vi "strange cluster.vi"(8 "Array In":T1(array[cluster]) {"Gauge" scale=0.0..100.0}, 11 "Cluster In":T2={"Gauge"=49.62882071738944, "Boolean def on"=TRUE, "My String"="abc", "Boolean def off"=FALSE, "Table"=[["1", "2", "3"], ["a", "b", "b"]], "Waveform Graph"={"t0"=timestamp(0 s since 1904-01-01), "dt"=0.001, "Y"=[0.0, 0.0634175857813252, 0.1265798623799041, 0.18923254844743084, 0.2511234141665813, 0.3120032966884148, 0.3716271032226454, 0.4297547977425003, 0.4861523673318466, 0.5405927642842268, 0.5928568201610591, 0.6427341281291522, 0.6900238900253773, 0.7345357247383564, 0.7760904346527414, 0.8145207270705094, 0.8496718877049362, 0.8814024035358785, 0.9095845325188363, 0.9341048178542484, 0.9548645447466428, 0.9717801378148127, 0.9847834975530967, 0.993822274489234, 0.9988600799350685, 0.9998766324816606, 0.9968678396490348, 0.9898458143618585, 0.9788388261847202, 0.9638911875133281, 0.9450630751798048, 0.9224302881902667, 0.8960839425699989, 0.8661301045447303, 0.8326893635347631, 0.7958963466810159, 0.7558991768574196, 0.7128588763516256, 0.6669487186147105, 0.6183535306896335, 0.5672689491267566, 0.5139006323819968, 0.458463432868368, 0.40118053199410575, 0.3422825416695715, 0.28200657590012973, 0.22059529620261753, 0.15829593468840908, 0.09535929874598903, 0.03203876133002422, -0.03141075907812785, -0.09473382473195789, -0.15767550697182214, -0.21998241252745737, -0.2814037036392598, -0.3416921078914828, -0.40060491369192236, -0.45790494739044835, -0.5133615281026551, -0.5667513963946633, -0.6178596130903338, -0.6664804245824388, -0.7124180911641828, -0.7554876750463428, -0.7955157848875944, -0.832341273840663, -0.8658158883040745, -0.8958048647677382, -0.9221874723495489, -0.944857498838849, -0.9637236782900093, -0.9787100584447116, -0.9897563065037406, -0.9968179520173057, -0.9998665659160451, -0.9988898749619699, -0.99389181115858, -0.9848924959212413, -0.9719281590715428, -0.9550509929817614, -0.934328942456612, -0.9098454311981998, -0.8816990259553703, -0.8500030397095515, -0.8148850754945864, -0.776486512687079, -0.7349619378353532, -0.6904785223184312, -0.6432153493404656, -0.593362692970051, -0.5411212521268765, -0.48670134259958137, -0.43032205034760956, -0.3722103494957459, -0.312600188572142, -0.251731548668498, -0.18984947731409485, -0.1272031019531499, -0.06404462699707955, -0.0006283184893772641], "attributes"=variant("NI_ChannelName"=variant(string "Sine"), "NI_ExpIsRelativeTime"=variant(bool TRUE), "NI_ExpStartTimeStamp"=variant(timestamp timestamp(3210167528.3009996 s since 1904-01-01)), "NI_ExpTimeStamp"=variant(timestamp timestamp(3210167528.3009996 s since 1904-01-01)), "NI_ExpXDimension"=variant(string "t"))}} {"Gauge" scale=0.0..100.0}) -> (0 "Array Out":T1(array[cluster]) {"Gauge" scale=0.0..100.0}, 3 "Cluster Out":T2={"Gauge"=49.62882071738944, "Boolean def on"=TRUE, "My String"="abc", "Boolean def off"=FALSE, "Table"=[["1", "2", "3"], ["a", "b", "b"]], "Waveform Graph"={"t0"=timestamp(0 s since 1904-01-01), "dt"=0.001, "Y"=[0.0, 0.0634175857813252, 0.1265798623799041, 0.18923254844743084, 0.2511234141665813, 0.3120032966884148, 0.3716271032226454, 0.4297547977425003, 0.4861523673318466, 0.5405927642842268, 0.5928568201610591, 0.6427341281291522, 0.6900238900253773, 0.7345357247383564, 0.7760904346527414, 0.8145207270705094, 0.8496718877049362, 0.8814024035358785, 0.9095845325188363, 0.9341048178542484, 0.9548645447466428, 0.9717801378148127, 0.9847834975530967, 0.993822274489234, 0.9988600799350685, 0.9998766324816606, 0.9968678396490348, 0.9898458143618585, 0.9788388261847202, 0.9638911875133281, 0.9450630751798048, 0.9224302881902667, 0.8960839425699989, 0.8661301045447303, 0.8326893635347631, 0.7958963466810159, 0.7558991768574196, 0.7128588763516256, 0.6669487186147105, 0.6183535306896335, 0.5672689491267566, 0.5139006323819968, 0.458463432868368, 0.40118053199410575, 0.3422825416695715, 0.28200657590012973, 0.22059529620261753, 0.15829593468840908, 0.09535929874598903, 0.03203876133002422, -0.03141075907812785, -0.09473382473195789, -0.15767550697182214, -0.21998241252745737, -0.2814037036392598, -0.3416921078914828, -0.40060491369192236, -0.45790494739044835, -0.5133615281026551, -0.5667513963946633, -0.6178596130903338, -0.6664804245824388, -0.7124180911641828, -0.7554876750463428, -0.7955157848875944, -0.832341273840663, -0.8658158883040745, -0.8958048647677382, -0.9221874723495489, -0.944857498838849, -0.9637236782900093, -0.9787100584447116, -0.9897563065037406, -0.9968179520173057, -0.9998665659160451, -0.9988898749619699, -0.99389181115858, -0.9848924959212413, -0.9719281590715428, -0.9550509929817614, -0.934328942456612, -0.9098454311981998, -0.8816990259553703, -0.8500030397095515, -0.8148850754945864, -0.776486512687079, -0.7349619378353532, -0.6904785223184312, -0.6432153493404656, -0.593362692970051, -0.5411212521268765, -0.48670134259958137, -0.43032205034760956, -0.3722103494957459, -0.312600188572142, -0.251731548668498, -0.18984947731409485, -0.1272031019531499, -0.06404462699707955, -0.0006283184893772641], "attributes"=variant("NI_ChannelName"=variant(string "Sine"), "NI_ExpIsRelativeTime"=variant(bool TRUE), "NI_ExpStartTimeStamp"=variant(timestamp timestamp(3210167528.3009996 s since 1904-01-01)), "NI_ExpTimeStamp"=variant(timestamp timestamp(3210167528.3009996 s since 1904-01-01)), "NI_ExpXDimension"=variant(string "t"))}} {"Gauge" scale=0.0..100.0})   [LabVIEW 2011]
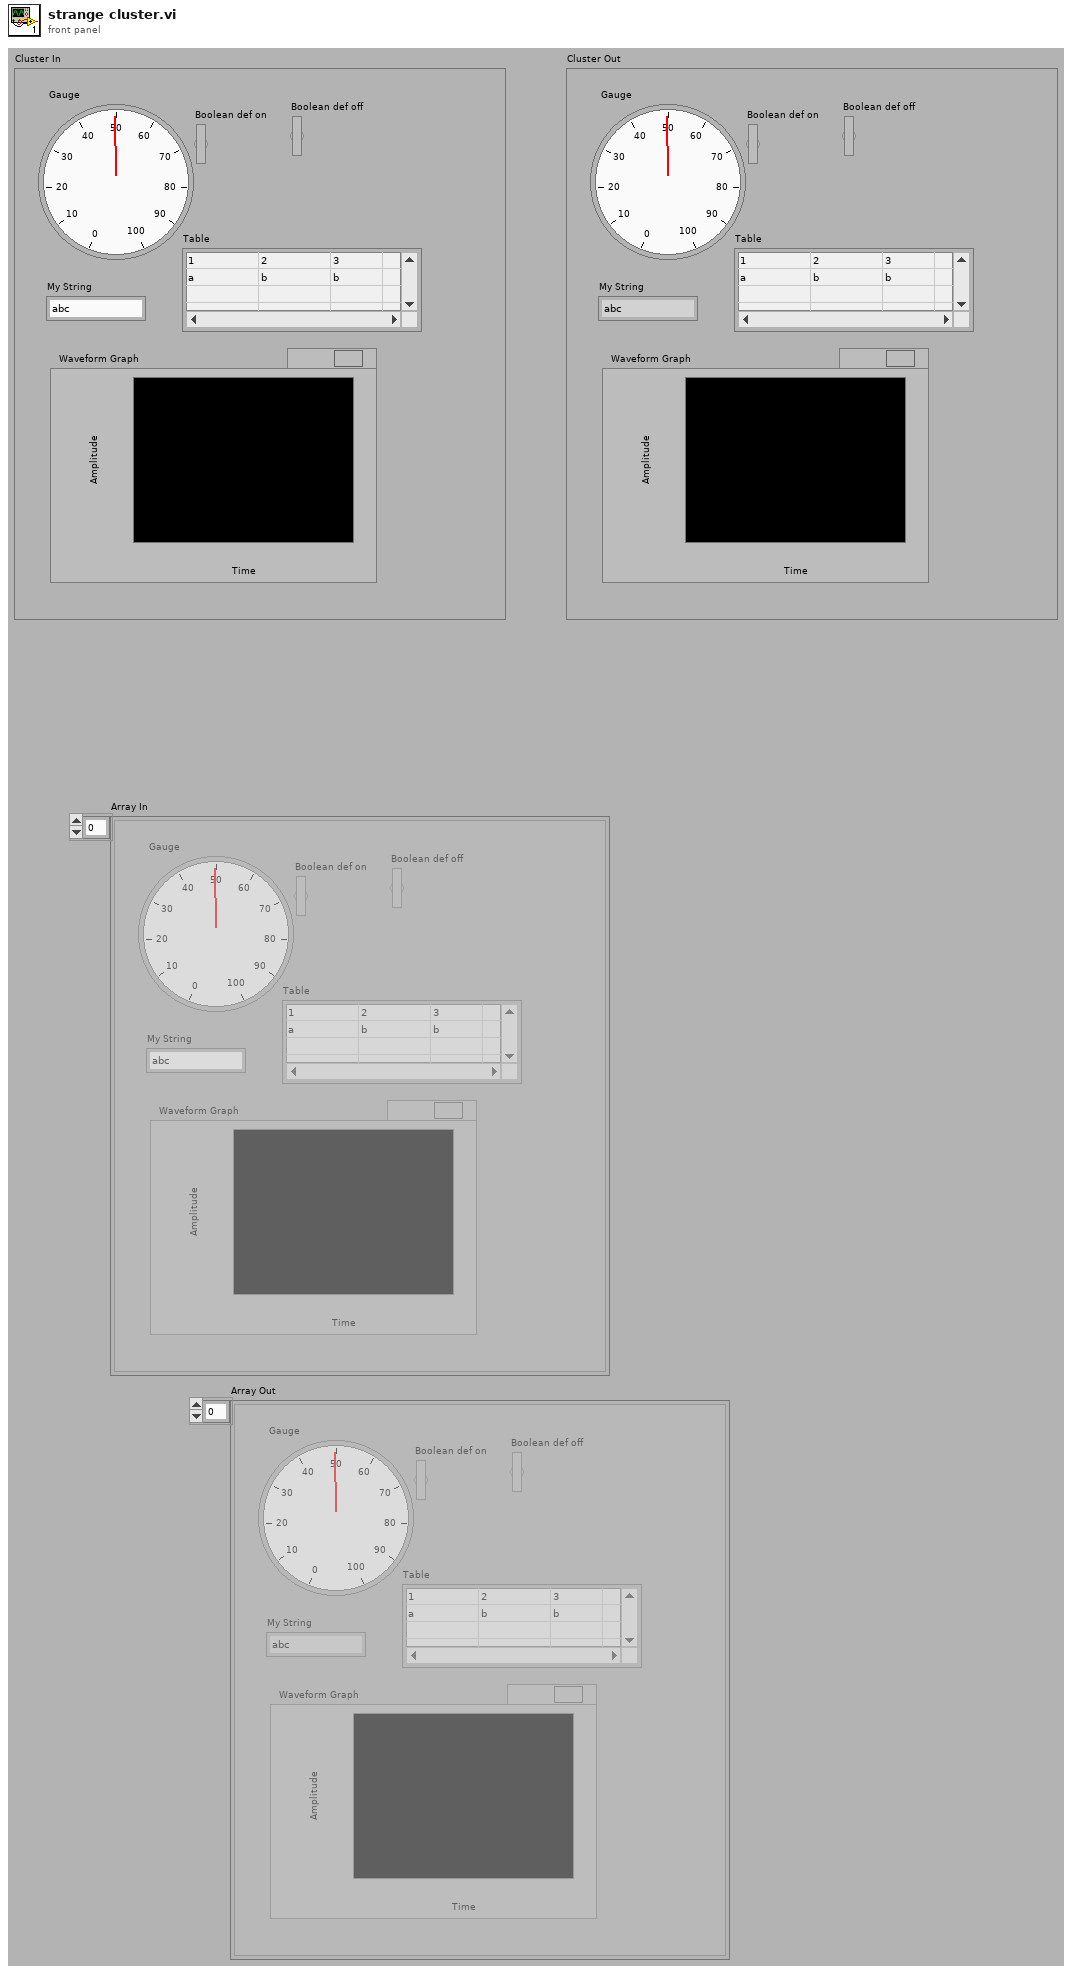
[diagram p1: front panel]
types:
  T1 = cluster{"Gauge":dbl, "Boolean def on":bool, "My String":string, "Boolean def off":bool, "Table":string[][], "Waveform Graph":waveform(dbl)}[]
  T2 = cluster{"Gauge":dbl, "Boolean def on":bool, "My String":string, "Boolean def off":bool, "Table":string[][], "Waveform Graph":waveform(dbl)}
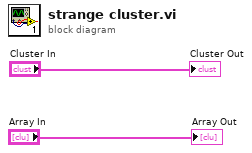
[diagram p0: block diagram]
diagram:
  "Cluster Out" <- "Cluster In"
  "Array Out" <- "Array In"
